vi "Reflection Point.vi"(5 "Parsed Formula":cluster{"Table":i32[][], "Y Values":dbl[]}, 6 "high index":u32=1, 7 "factor":dbl format="%.2f", 8 "f values before":dbl[](array[numeric]) format="%.2f", 9 "psum before":dbl[](array[numeric]) format="%.2f", 10 "Variables":i32[](array[numeric]), 11 "points before":dbl[][](array[numeric]) format="%.2f") -> (0 "f values after":dbl[](array[numeric]) format="%.2f", 1 "psum after":dbl[](array[numeric]) format="%.2f", 3 "points after":dbl[][](array[numeric]) format="%.2f", 4 "new f value":dbl format="%.2f")   [LabVIEW 2018, in "NI_Gmath.lvlib"]
uses:
  NI_Gmath.lvlib
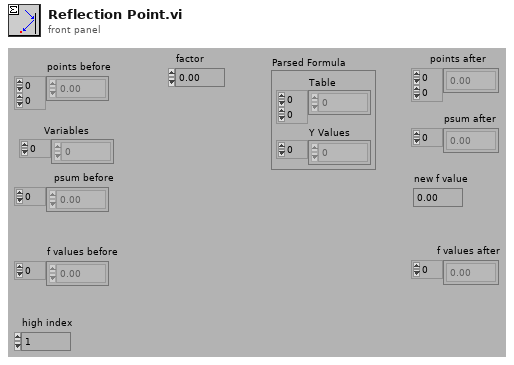
[diagram p1: front panel]
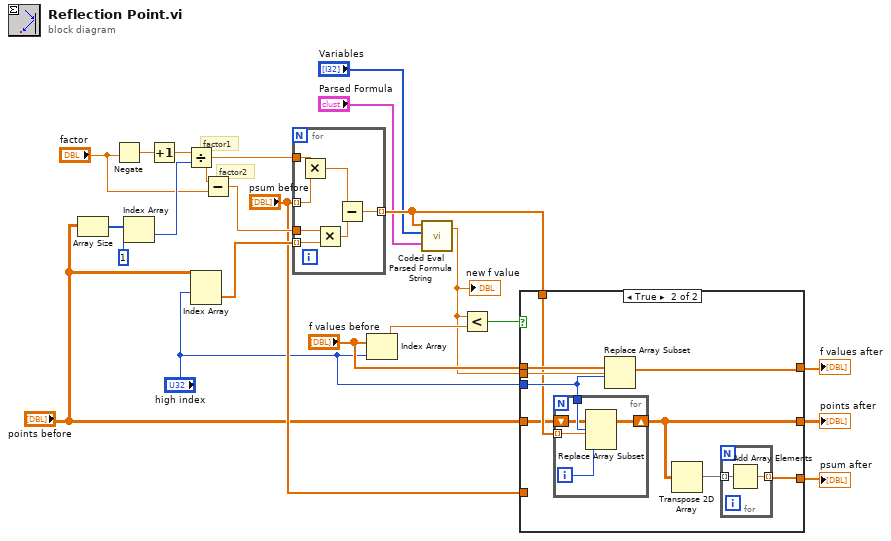
[diagram p0: block diagram]
diagram:
  # "factor2"
  # "factor1"
  n1 = Array Size(array="points before") -> (size(s)=w22:i32[])
  n2 = Negate(x="factor") -> (-x=w20:dbl)
  n3 = Index Array(array=w22, index=1) -> (element=w18:i32)
  n4 = Increment(x=w20) -> (x+1=w19:dbl)
  n5 = Divide(x=w19, y=w18) -> (x/y=w17:dbl)
  n6 = Index Array(array="points before", index (row)="high index") -> (element=w15:dbl[])  [unwired: 1 in]
  n7 = Subtract(x=w17, y="factor") -> (x-y=w14:dbl)
  n8 = for {
    tunnel: w17 -> [w29]
    tunnel: "psum before" -> [w28] mode=indexing
    tunnel: w15 -> [w27] mode=indexing
    tunnel: w14 -> [w26]
    tunnel: [w23] -> w4 mode=indexing
    n9 = Multiply(x=w29, y=w28) -> (x*y=w25:dbl)
    n10 = Multiply(x=w26, y=w27) -> (x*y=w24:dbl)
    n11 = Subtract(x=w25, y=w24) -> (x-y=w23:dbl)
  }
  n12 = Index Array(array="f values before", index="high index") -> (element=w9:dbl)
  n13 = call "Coded Eval Parsed Formula String.vi"("Parsed Formula"="Parsed Formula", "Variables"="Variables", "X Values"=w4) -> ("y value"=w3:dbl)  [unwired: 1 in, 1 out]
  "new f value" <- w3
  n14 = Less?(x=w3, y=w9) -> (x < y?=w5:bool)
  n15 = case shown="True" w5 {
    tunnel: "psum before" -> [w32 _]
    tunnel: [w32 w35] -> w12
    tunnel: "points before" -> [w31 w34]
    tunnel: [w31 w33] -> w10
    tunnel: "f values before" -> [w30 w41]
    tunnel: [w30 w39] -> w7
    tunnel: "high index" -> [_ w38]
    tunnel: w3 -> [_ w40]
    tunnel: w4 -> [_ w37]
    frame False {
    }
    frame True {
      n16 = for {
        tunnel: w38 -> [w47]
        tunnel: w37 -> [w46] mode=indexing
        shift-right: [w44] -> w33
        shift-left: w34 -> [w45]
        i -> [w48]
        n17 = Replace Array Subset(array=w45, new element=w46, index (row)=w47, index (col)=w48) -> (w44:dbl[][])
      }
      n18 = Replace Array Subset(array=w41, new element=w40, index=w38) -> (w39:dbl[])
      n19 = Transpose 2D Array(2D array=w33) -> (transposed array=w36:dbl[][])
      n20 = for {
        tunnel: w36 -> [w43] mode=indexing
        tunnel: [w42] -> w35 mode=indexing
        n21 = Add Array Elements(numeric array=w43) -> (sum=w42:dbl)
      }
    }
  }
  "points after" <- w10
  "psum after" <- w12
  "f values after" <- w7
